vi "Change Fixed.vi"(2 "Locked Traces":bool[](array[boolean])=[FALSE, FALSE, FALSE, FALSE, FALSE, FALSE, FALSE, FALSE, FALSE, TRUE], 4 "Trace Names":string[](array[string])=["Current", "Previous", "older", "Ref#1", "Ref#2", "Ref#3", "Ref#4", "Ref#5", "Ref#6", "Ref#7"] caption="Column Headings") -> (0 "StoreInto output":u16(ring) items=["Store Into", "previous", "older", "Ref#1", "Ref#2", "Ref#3", "Ref#4", "Ref#5", "Ref#6", "Ref#77"], 1 "Pin output":bool[](array[boolean])=[FALSE, FALSE, FALSE, FALSE, FALSE, FALSE, FALSE, FALSE, FALSE, TRUE])   [LabVIEW 2019]
panel:
  out "String":string
  in  "StoreInto":u16(ring) items=["Current", "previous", "older", "Ref#1", "Ref#2222", "Ref#3", "Ref#4", "Ref#5", "Ref#6", "Ref#77"]
  in  "quit":bool
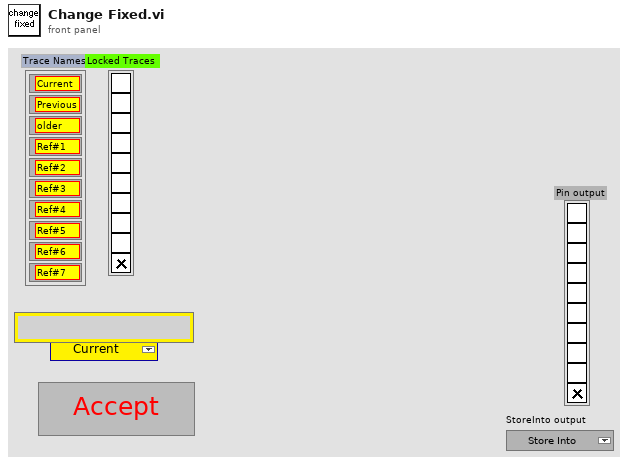
[diagram p1: front panel]
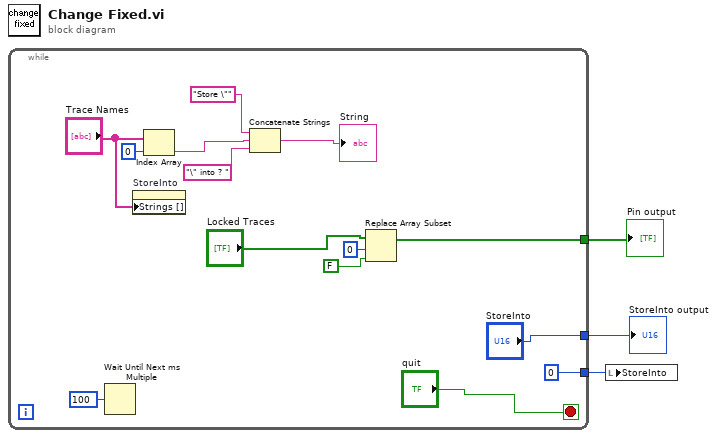
[diagram p0: block diagram]
diagram:
  n1 = while {
    tunnel: [w12] -> w3
    tunnel: ["StoreInto"] -> w2
    tunnel: [0 ("index")] -> w1
    stop <- "quit" stop-if-true
    n2 = Wait Until Next ms Multiple(millisecond multiple=u32 100) -> ()  [unwired: 1 out]
    n3 = property on="StoreInto" class="Ring (strict)"("Strings []"="Trace Names") -> ()  [unwired: 2 in, 2 out]
    n4 = Index Array(array="Trace Names", index=0) -> (element=w9:string)
    n5 = Concatenate Strings("Store \"", w9, "\" into ? ") -> (→"String":string)
    n6 = Replace Array Subset(array="Locked Traces", new element=FALSE ("new element/subarray"), index=0) -> (w12:bool[])
  }
  "Pin output" <- w3
  "StoreInto output" <- w2
  n7 = local write "StoreInto"(w1) -> ()
